vi "Send Query.vi"(8 "error in (no error)":errorcluster, 9 "byte count (1024)":u32=1024, 10 "write buffer":string, 11 "VISA resource name":refnum<visa-resource-name>) -> (0 "error out":errorcluster, 1 "return count":u32, 2 "read buffer":string, 3 "VISA resource name out":refnum<visa-resource-name>)   [LabVIEW 2023, in "Tektronix AFG 3000 Series.lvlib"]
doc: "Acquires a lock on the specified AFG3000 series function generator, sends the given query, reads the specified number of bytes, and checks for errors."
uses:
  Tektronix AFG 3000 Series.lvlib
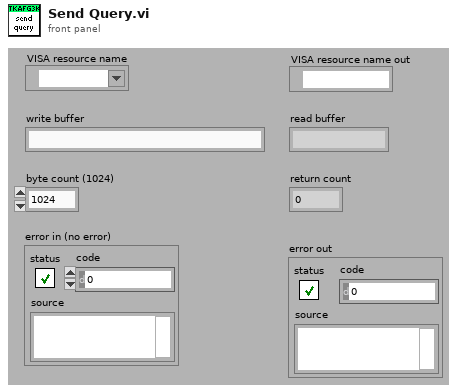
[diagram p1: front panel]
types:
  T1 = typedef "Semaphore RefNum" = refnum<k1>
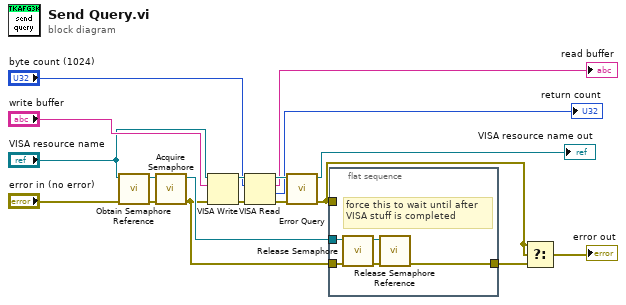
[diagram p0: block diagram]
diagram:
  n1 = call <vilib>:"Obtain Semaphore Reference.vi"("error in (no error)"="error in (no error)", "name (unnamed)"="VISA resource name") -> ("error out"=w10:errorcluster, "semaphore"=w9:T1)  [unwired: 1 in, 3 out]
  n2 = call <vilib>:"Acquire Semaphore.vi"("error in (no error)"=w10, "semaphore"=w9) -> ("error out"=w2:errorcluster, "semaphore out"=w6:T1)  [unwired: 1 in, 3 out]
  n3 = VISA Write(VISA resource name="VISA resource name", write buffer="write buffer", error in (no error)=w2) -> (VISA resource name out=w17:refnum<visa-resource-name>, error out=w16:errorcluster)  [unwired: 1 out]
  n4 = VISA Read(VISA resource name=w17, byte count="byte count (1024)", error in (no error)=w16) -> (VISA resource name out=w14:refnum<visa-resource-name>, read buffer=→"read buffer":string, return count=→"return count":u32, error out=w15:errorcluster)
  n5 = call "Error Query.vi"("error in (no error)"=w15, "VISA resource name"=w14) -> ("error out"=w1:errorcluster, "VISA resource name out"=→"VISA resource name out":refnum<visa-resource-name>)  [unwired: 8 out]
  n6 = flat-sequence {
    tunnel: w6 -> [w21]
    tunnel: w2 -> [w20]
    tunnel: [w19] -> w3
    tunnel: w1 -> [_]
    frame #0 {
      # "force this to wait until after \nVISA stuff is completed"
      n7 = call <vilib>:"Release Semaphore.vi"("error in (no error)"=w20, "semaphore"=w21) -> ("error out"=w22:errorcluster, "semaphore out"=w23:T1)  [unwired: 4 out]
      n8 = call <vilib>:"Release Semaphore Reference.vi"("error in (no error)"=w22, "semaphore"=w23) -> ("error out"=w19:errorcluster)  [unwired: 9 out]
    }
  }
  n9 = Select(t=w1, s=w1, f=w3) -> (s? t:f=→"error out":errorcluster)
